vi "MB Update Registers.vi"(8 "error in (no error)":errorcluster, 10 "Data Reference":T1, 11 "Modbus Data Unit In":T2={"function"=1, "Data"=[]} {"function" items=["Read Discrete Inputs"=2, "Read Coils"=1, "Write Single Coil"=5, "Write Multiple Coils"=15, "Read Input Register"=4, "Read Holding Registers"=3, "Write Single Register"=6, "Write Multiple Registers"=16, "Read/Write Multiple Registers"=23, "Mask Write Register"=22, "Read FIFO Queue"=24, "Read File Record"=20, "Write File Record"=21, "Read Exception Status"=7, "Diagnostic"=8, "Get Com Event Counter"=11, "Get Com Event Log"=12, "Report Slave ID"=17, "Read Device Identification"=43]; "Data" format="%.0x"}) -> (0 "error out":errorcluster, 3 "Modbus Data Unit Out":T2={"function"=1, "Data"=[]} {"function" items=["Read Discrete Inputs"=2, "Read Coils"=1, "Write Single Coil"=5, "Write Multiple Coils"=15, "Read Input Register"=4, "Read Holding Registers"=3, "Write Single Register"=6, "Write Multiple Registers"=16, "Read/Write Multiple Registers"=23, "Mask Write Register"=22, "Read FIFO Queue"=24, "Read File Record"=20, "Write File Record"=21, "Read Exception Status"=7, "Diagnostic"=8, "Get Com Event Counter"=11, "Get Com Event Log"=12, "Report Slave ID"=17, "Read Device Identification"=43]; "Data" format="%.0x"})   [LabVIEW 2019, in "NI_modbus_upd.lvlib"]
uses:
  NI_modbus_upd.lvlib
  MB Globals.vi
  Standard Data Model/Standard Data Model1.lvclass
  Ctl/MB Modbus Data Unit.ctl
  Ctl/Data Reference.ctl
  Modbus Data Unit (PDU)/Function.ctl
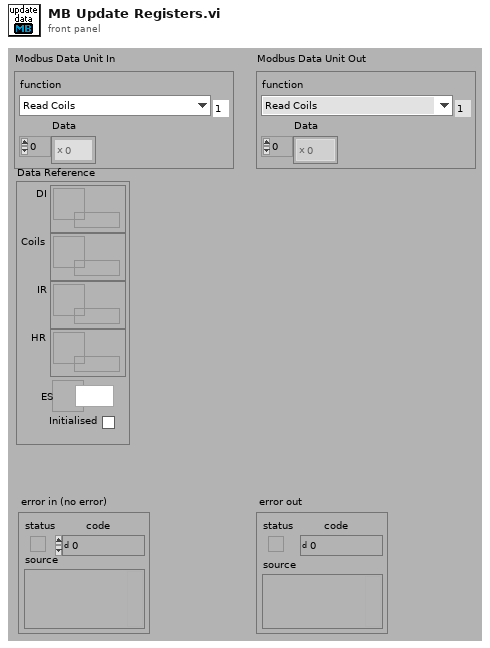
[diagram p1: front panel]
types:
  T1 = typedef "NI_modbus_upd.lvlib/Data Reference.ctl" = cluster{"DI":refnum<data-value>, "Coils":refnum<data-value>, "IR":refnum<data-value>, "HR":refnum<data-value>, "ES":refnum<data-value>, "Initialised":bool}
  T2 = typedef "NI_modbus_upd.lvlib/MB Modbus Data Unit.ctl" = cluster{"function":T3, "Data":u8[]}
  T3 = typedef "NI_modbus_upd.lvlib/Function.ctl" = u8
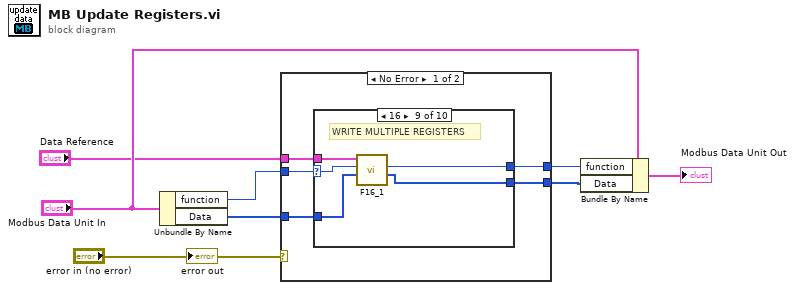
[diagram p0: block diagram]
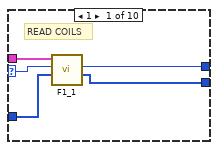
[diagram p2: hidden frame]
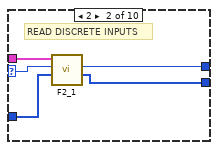
[diagram p3: hidden frame]
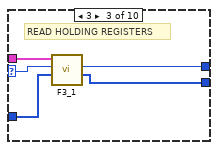
[diagram p4: hidden frame]
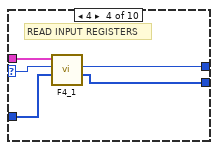
[diagram p5: hidden frame]
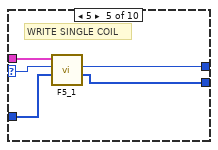
[diagram p6: hidden frame]
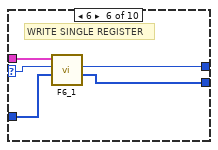
[diagram p7: hidden frame]
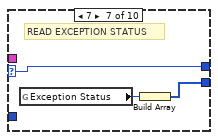
[diagram p8: hidden frame]
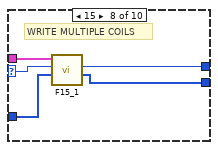
[diagram p9: hidden frame]
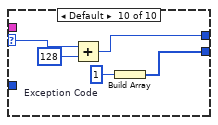
[diagram p10: hidden frame]
diagram:
  n1 = Unbundle By Name("Modbus Data Unit In") -> ("function"=w2:T3, "Data"=w1:u8[])
  n2 = case shown="No Error" "error in (no error)" {
    tunnel: [w13 w63] -> w7
    tunnel: w1 -> [w12 w63]
    tunnel: w2 -> [w11 w62]
    tunnel: [w10 w62] -> w5
    tunnel: "Data Reference" -> [w9 _]
    frame No Error {
      n3 = case shown="16" w11 {
        selector: w11 -> [w17 w22 w27 w32 w37 w39 w45 w50 w55 w60]
        tunnel: w12 -> [w16 w21 w26 w31 w36 w40 _ w49 w54 _]
        tunnel: [w14 w19 w24 w29 w34 w41 w46 w47 w52 w59] -> w13
        tunnel: [w15 w20 w25 w30 w35 w42 w45 w48 w53 w58] -> w10
        tunnel: w9 -> [w18 w23 w28 w33 w38 w43 _ w51 w56 _]
        frame 1 {
          # "READ COILS"
          n4 = call "F1_1.vi"("data"=w16, "function"=w17, "device data model in"=w18) -> ("data return"=w14:u8[], "function return"=w15:u8)  [unwired: 5 in, 2 out]
        }
        frame 2 {
          # "READ DISCRETE INPUTS"
          n5 = call "F2_1.vi"("data"=w21, "function"=w22, "device data model in"=w23) -> ("data return"=w19:u8[], "function return"=w20:u8)  [unwired: 5 in, 2 out]
        }
        frame 3 {
          # "READ HOLDING REGISTERS"
          n6 = call "F3_1.vi"("data"=w26, "function"=w27, "device data model in"=w28) -> ("data return"=w24:u8[], "function return"=w25:u8)  [unwired: 5 in, 2 out]
        }
        frame 4 {
          # "READ INPUT REGISTERS"
          n7 = call "F4_1.vi"("data"=w31, "function"=w32, "device data model in"=w33) -> ("data return"=w29:u8[], "function return"=w30:u8)  [unwired: 5 in, 2 out]
        }
        frame 5 {
          # "WRITE SINGLE COIL"
          n8 = call "F5_1.vi"("data"=w36, "function"=w37, "device data model in"=w38) -> ("data return"=w34:u8[], "function return"=w35:u8)  [unwired: 5 in, 2 out]
        }
        frame 6 {
          # "WRITE SINGLE REGISTER"
          n9 = call "F6_1.vi"("data"=w40, "function"=w39, "device data model in"=w43) -> ("data return"=w41:u8[], "function return"=w42:u8)  [unwired: 5 in, 2 out]
        }
        frame 7 {
          # "READ EXCEPTION STATUS"
          n10 = global read "MB Globals.vi" "Exception Status"() -> (w44:u8)
          n11 = Build Array(w44) -> (w46:u8[])
        }
        frame 15 {
          # "WRITE MULTIPLE COILS"
          n12 = call "F15_1.vi"("data"=w49, "function"=w50, "device data model in"=w51) -> ("data return"=w47:u8[], "function return"=w48:u8)  [unwired: 5 in, 2 out]
        }
        frame 16 {
          # "WRITE MULTIPLE REGISTERS"
          n13 = call "F16_1.vi"("data"=w54, "function"=w55, "device data model in"=w56) -> ("data return"=w52:u8[], "function return"=w53:u8)  [unwired: 5 in, 2 out]
        }
        frame Default {
          w57 = u8 1  # Exception Code
          n14 = Add(x=w60, y=u8 128) -> (x+y=w58:T3)
          n15 = Build Array(w57) -> (w59:u8[])
        }
      }
    }
    frame Error {
    }
  }
  n16 = Bundle By Name(cluster="Modbus Data Unit In", "function"=w5, "Data"=w7) -> (→"Modbus Data Unit Out":T2)
  "error out" <- "error in (no error)"
